vi "Windows Popup Menu.vi"() -> ()   [LabVIEW 2020]
uses:
  <vilib>/Utility/miscctls.llb/LVPointTypeDef.ctl
  user32.dll
  kernel32.dll
panel:
  in  "Open Menu":bool
  out "Append Bool":i32
  out "Window Handle Match":bool
  out "hMenu":u64
  out "TrackPop Bool":i32
  out "Destory Bool":i32
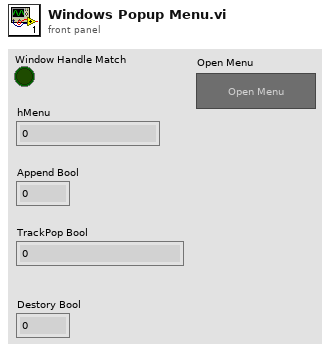
[diagram p1: front panel]
types:
  T1 = typedef "LVPointTypeDef.ctl" = cluster{"Horizontal":i16, "Vertical":i16}
  T2 = typedef "LVPositionTypeDef.ctl" = cluster{"Left":i32, "Top":i32}
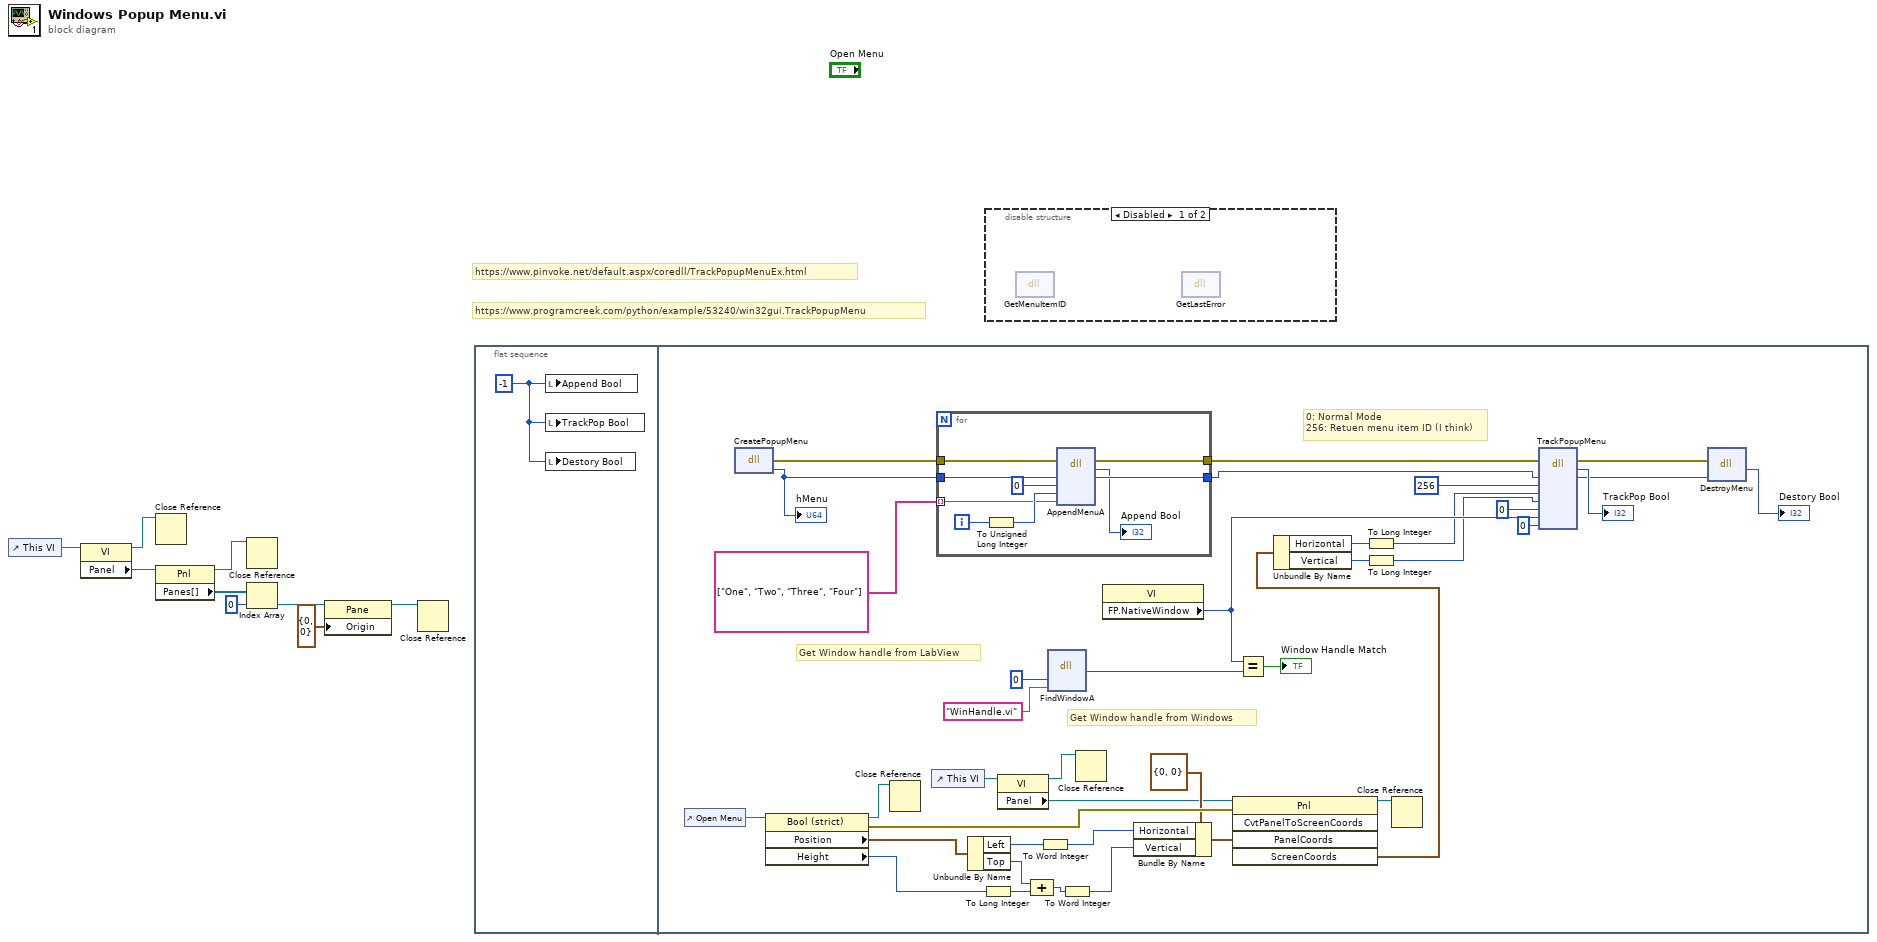
[diagram p0: block diagram]
diagram:
  # "https://www.programcreek.com/python/example/53240/win32gui.TrackPopupMenu"
  # "https://www.pinvoke.net/default.aspx/coredll/TrackPopupMenuEx.html"
  n1 = control-ref of="This VI"() -> (w9:refnum<vi>)
  n2 = property class="VI"(reference=w9) -> (reference out=w1:refnum<vi>, "Panel"=w8:refnum<vi>)  [unwired: 1 in, 1 out]
  n3 = Close Reference(reference=w1) -> ()  [unwired: 1 in, 1 out]
  n4 = property class="Pnl"(reference=w8) -> (reference out=w2:refnum<vi>, "Panes[]"=w7:refnum<vi>[])  [unwired: 1 in, 1 out]
  n5 = Close Reference(reference=w2) -> ()  [unwired: 1 in, 1 out]
  n6 = Index Array(array=w7, index=0) -> (element=w5:refnum<vi>)
  n7 = property class="Pane"(reference=w5, "Origin"=T1 {"Horizontal"=0, "Vertical"=0}) -> (reference out=w3:refnum<vi>)  [unwired: 1 in, 1 out]
  n8 = Close Reference(reference=w3) -> ()  [unwired: 1 in, 1 out]
  n9 = flat-sequence {
    frame #0 {
      w10 = -1 ("Append Bool")
      n10 = local write "Append Bool"(w10) -> ()
      n11 = local write "TrackPop Bool"(w10) -> ()
      n12 = local write "Destory Bool"(w10) -> ()
    }
    frame #1 {
      # "Get Window handle from Windows"
      # "Get Window handle from LabView"
      # "0: Normal Mode\n256: Retuen menu item ID (I think)"
      n13 = control-ref of="Open Menu"() -> (w17:refnum<vi>)
      n14 = dll-call lib="user32.dll" fn="CreatePopupMenu"() -> (error out=w48:errorcluster, "hMenu"=w47:u64)  [unwired: 3 in, 1 out]
      "hMenu" <- w47
      n15 = property on="Property Node" class="Bool (strict)"(reference=w17) -> (reference out=w18:refnum<vi>, error out=w32:errorcluster, "Position"=w22:T2, "Height"=w27:u32)  [unwired: 1 in]
      n16 = Close Reference(reference=w18) -> ()  [unwired: 1 in, 1 out]
      n17 = control-ref of="This VI"() -> (w16:refnum<vi>)
      n18 = for {
        tunnel: w48 -> [w56]
        tunnel: w47 -> [w55]
        tunnel: string[] ["One", "Two", "Three", "Four"] -> [w53] mode=indexing
        tunnel: [w52] -> w37
        tunnel: [w51] -> w36
        i -> [w58]
        n19 = To Unsigned Long Integer(number=w58) -> (unsigned 32bit integer=w54:u32)
        n20 = dll-call lib="user32.dll" fn="AppendMenuA"(error in=w56, "hMenu"=w55, "uFlags"=u32 0, "uIDNewItem"=w54, "lpNewItem"=w53) -> (error out=w52:errorcluster, "BOOL"=→"Append Bool":i32, "hMenu"=w51:u64)  [unwired: 5 in, 1 out]
      }
      n21 = Unbundle By Name(w22) -> ("Left"=w29:i32, "Top"=w23:i32)
      n22 = To Long Integer(number=w27) -> (32bit integer=w25:i32)
      n23 = property class="VI"(reference=w16) -> (reference out=w19:refnum<vi>, "Panel"=w21:refnum<vi>)  [unwired: 1 in, 1 out]
      n24 = Compound Arithmetic op=ADD(w23, w25) -> (w24:i32)
      n25 = To Word Integer(number=w29) -> (16bit integer=w28:i16)
      n26 = dll-call lib="user32.dll" fn="FindWindowA"("lpClassName"=u8 0, "lpWindowName"="WinHandle.vi") -> ("hWnd"=w45:u64)  [unwired: 5 in, 2 out]
      n27 = To Word Integer(number=w24) -> (16bit integer=w26:i16)
      n28 = Close Reference(reference=w19) -> ()  [unwired: 1 in, 1 out]
      n29 = property class="VI"() -> ("FP.NativeWindow"=w43:u64)  [unwired: 2 in, 2 out]
      n30 = Bundle By Name(cluster=T1 {"Horizontal"=0, "Vertical"=0} ("Panel Coordinates"), "Horizontal"=w28, "Vertical"=w26) -> (w30:T1)
      n31 = invoke class="Pnl" method="CvtPanelToScreenCoords"(reference=w21, error in=w32, "PanelCoords"=w30) -> (reference out=w20:refnum<vi>, "ScreenCoords"=w13:T1)  [unwired: 2 in, 3 out]
      n32 = Equal?(x=w43, y=w45) -> (x = y?=→"Window Handle Match":bool)
      n33 = Unbundle By Name(w13) -> ("Horizontal"=w15:i16, "Vertical"=w14:i16)
      n34 = To Long Integer(number=w15) -> (32bit integer=w12:i32)
      n35 = To Long Integer(number=w14) -> (32bit integer=w11:i32)
      n36 = Close Reference(reference=w20) -> ()  [unwired: 1 in, 1 out]
      n37 = dll-call lib="user32.dll" fn="TrackPopupMenu"(error in=w37, "hMenu"=w36, "uFlags"=u32 256, "x"=w12, "y"=w11, "nReserved"=0, "hwnd"=w43, "prcRect"=u64 0) -> (error out=w34:errorcluster, "BOOL"=→"TrackPop Bool":i32, "hMenu"=w33:u64)  [unwired: 8 in, 1 out]
      n38 = dll-call lib="user32.dll" fn="DestroyMenu"(error in=w34, "hMenu"=w33) -> ("BOOL"=→"Destory Bool":i32)  [unwired: 3 in, 2 out]
    }
  }
  n39 = disable-structure shown="Disabled" {
    frame Disabled {
      n40 = dll-call lib="user32.dll" fn="GetMenuItemID"() -> ()  [unwired: 4 in, 2 out]
      n41 = dll-call lib="kernel32.dll" fn="GetLastError"() -> ()  [unwired: 4 in, 2 out]
    }
    frame Enabled {
    }
  }
